vi "Shared Variable Initialization VI.vi"(8 "error in (no error)":errorcluster, 10 "Custom XML":string, 11 "Device Item Ref in":T1 format="%.0x") -> (0 "error out":errorcluster, 3 "Device Item Ref out":T1 format="%.0x")   [LabVIEW 2012, in "Shared Variable Custom Device.lvlib"]
uses:
  Shared Variable Custom Device.lvlib
  <vilib>/NI Veristand/Custom Device API/Custom Device Item Ref.ctl
  <vilib>/NI Veristand/Custom Device API/Custom Device Channel.ctl
  <vilib>/NI Veristand/Custom Device API/Custom Device Channel Type.ctl
  Shared/Shared Variable GUID Lookup.vi
  Shared/Shared Variable Globals.vi
  <vilib>/NI Veristand/Custom Device API/Custom Device API.lvlib
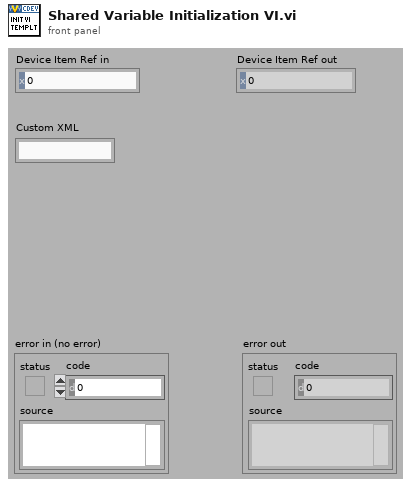
[diagram p1: front panel]
types:
  T1 = typedef "Custom Device API.lvlib/Custom Device Item Ref.ctl" = u64
  T2 = typedef "Custom Device API.lvlib/Custom Device Channel.ctl" = cluster{"Type":T3, "Units":string, "Default Value":dbl, "Faultable":bool, "Scalable":bool}
  T3 = typedef "Custom Device API.lvlib/Custom Device Channel Type.ctl" = enum16{"Input", "Output"}
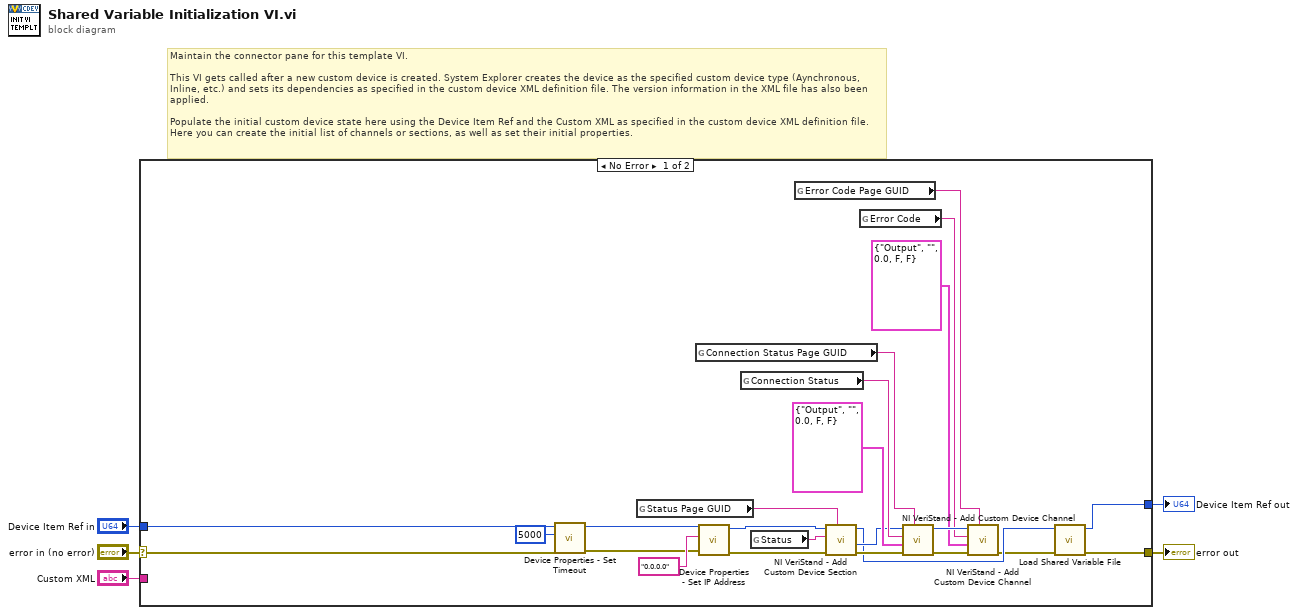
[diagram p0: block diagram]
diagram:
  # "Maintain the connector pane for this template VI.\n\nThis VI gets called after a new custom device is created. System Explorer creates the device as the specified custom device type (Aynchronous, Inline, etc.) and sets its dependencies as specified in the custom device XML definition file. The version information in the XML file has also been applied.\n\nPopulate the initial custom device state here using the Device Item Ref and the Custom XML as specified in the custom device XML definition file. Here you can create the initial list of channels or sections, as well as set their initial properties."
  n1 = case shown="No Error" "error in (no error)" {
    selector: "error in (no error)" -> [w12 w31]
    tunnel: [w6 w31] -> w5
    tunnel: [w8 w30] -> w3
    tunnel: "Device Item Ref in" -> [w14 w30]
    tunnel: "Custom XML" -> [_ _]
    frame No Error {
      n2 = call "Device Properties - Set Timeout.vi"("error in (no error)"=w12, "IP Address"=5000, "Device Ref in"=w14) -> ("error out"=w11:errorcluster, "Device Ref out"=w13:T1)  [unwired: 7 in]
      n3 = global read "Shared Variable GUID Lookup.vi" "Status Page GUID"() -> (w28:string)
      n4 = global read "Shared Variable GUID Lookup.vi" "Connection Status Page GUID"() -> (w19:string)
      n5 = call "Device Properties - Set IP Address.vi"("error in (no error)"=w11, "IP Address"="0.0.0.0", "Device Ref in"=w13) -> ("error out"=w15:errorcluster, "Device Ref out"=w16:T1)  [unwired: 7 in]
      n6 = global read "Shared Variable Globals.vi" "Connection Status"() -> (w25:string)
      n7 = global read "Shared Variable Globals.vi" "Status"() -> (w27:string)
      n8 = global read "Shared Variable GUID Lookup.vi" "Error Code Page GUID"() -> (w18:string)
      n9 = call <vilib>:"NI VeriStand - Add Custom Device Section.vi"("GUID (Default Section)"=w28, "error in (no error)"=w15, "Section Name"=w27, "Parent Ref in"=w16) -> ("error out"=w26:errorcluster, "Section Ptr"=w17:T1, "Parent Ref out"=w9:T1)  [unwired: 4 in, 1 out]
      n10 = global read "Shared Variable Globals.vi" "Error Code"() -> (w22:string)
      n11 = call <vilib>:"NI VeriStand - Add Custom Device Channel.vi"("GUID (Default Channel)"=w19, "error in (no error)"=w26, "Channel"=T2 {"Type"=enum."Output", "Units"="", "Default Value"=0.0, "Faultable"=FALSE, "Scalable"=FALSE}, "Channel Name"=w25, "Parent Ref in"=w17) -> ("error out"=w24:errorcluster, "Parent Ref out"=w23:T1)  [unwired: 3 in, 2 out]
      n12 = call <vilib>:"NI VeriStand - Add Custom Device Channel.vi"("GUID (Default Channel)"=w18, "error in (no error)"=w24, "Channel"=T2 {"Type"=enum."Output", "Units"="", "Default Value"=0.0, "Faultable"=FALSE, "Scalable"=FALSE}, "Channel Name"=w22, "Parent Ref in"=w23) -> ("error out"=w7:errorcluster)  [unwired: 3 in, 3 out]
      n13 = call "Load Shared Variable File.vi"("error in"=w7, "Device Ref in"=w9) -> ("error out"=w6:errorcluster, "Device Ref out"=w8:T1)  [unwired: 8 in]
    }
    frame Error {
    }
  }
  "error out" <- w5
  "Device Item Ref out" <- w3
